vi "TimeTag_LSW_edits_oct28.vi"() -> ()   [LabVIEW 2015]
doc: "This sample project is built upon the standard state machine template and shows how you could create an application that acquires, analyzes, and presents data. It includes functionality for presenting configuration dialogs, preserving settings between executions, loading and saving data, as well as exporting graph images and text files.\n\nIt is most appropriate for data that is acquired instantly as it does not allow for screen updates mid acquisition nor does it allow for continuous streaming to disk."
uses:
  <vilib>/ptbypt/NI_PtbyPt.lvlib
panel:
  out "Channel 2&4 counts/sec":T1(graph)
  out "real coin cps 100 sec avg":dbl
  out "all coin cps":dbl
  out "real coin cps":dbl
  out "random coin cps":dbl
  out "Real coin cps":dbl(graph)
  out "total coin/sec - total random coin/sec":dbl
  out "total random coincidences/sec":dbl
  out "Total Coin per sec":dbl
  out "Ch2/4 coin/sec":dbl(graph)
  out "Ch2/4 Total Coincidences":dbl
  out "Channel 2 CPS":dbl(graph)
  out "Channel 4 CPS":dbl(graph)
  out "Total Ch2 CPS":dbl
  out "Total Ch4 CPS":dbl
  in  "Averaging":dbl=10.0
  in  "Runs":dbl=100.0
  in  "Pulse TTL 2":bool
  in  "Pulse TTL 1":bool
  in  "Toggle\nTTL 2":bool
  in  "Toggle\nTTL 1":bool
  out "Total Starts":dbl
  in  "Record data":bool
  out "Initial time":dbl
  out "Elapsed time (s)":dbl
  out "FPGA_Run Status":dbl
  out "USB_Open Status":dbl
  out "Channel 4 Total\nCounts":dbl
  out "Channel 3 Total\nCounts":dbl
  out "Channel 2 Total\nCounts":dbl
  out "Channel 1 Total\nCounts":dbl
  in  "File Name":string="C:\\FPGA\\test.txt"
  out "?":dbl
  out "?":dbl
  out "?":dbl
  out "?":dbl
  out "stats":i64[](array[numeric])
  in  "Stop":bool
  out "Channel 4 CPS":dbl(knob) scale=0.0..2000000.0
  out "Channel 3 CPS":dbl(knob) scale=0.0..600.0
  out "Channel 2 CPS":dbl(knob) scale=0.0..700.0
  out "Channel 1 CPS":dbl(knob) scale=0.0..600.0
  # "Starts"
  # "Channel 1"
  # "Channel 2"
  # "Channel 3"
  # "Channel 4"
  # "Coincidence Channels 1 & 2"
  # "Coincidence Channels 1 & 3"
  # "Coincidence Channels 1 & 4"
  # "Coincidence Channels 2 & 3"
  # "Coincidence Channels 2 & 4"
  # "Coincidence Channels 3 & 4"
  # "Coincidence Channels 1 & 2 & 3"
  # "Coincidence Channels 1 & 2 & 4"
  # "Coincidence Channels 1 & 3 & 4"
  # "Coincidence Channels 2 & 3 & 4"
  # "C:\\FPGA_Lauren"
  # "Coincidence Channels 1 & 2 & 3 & 4"
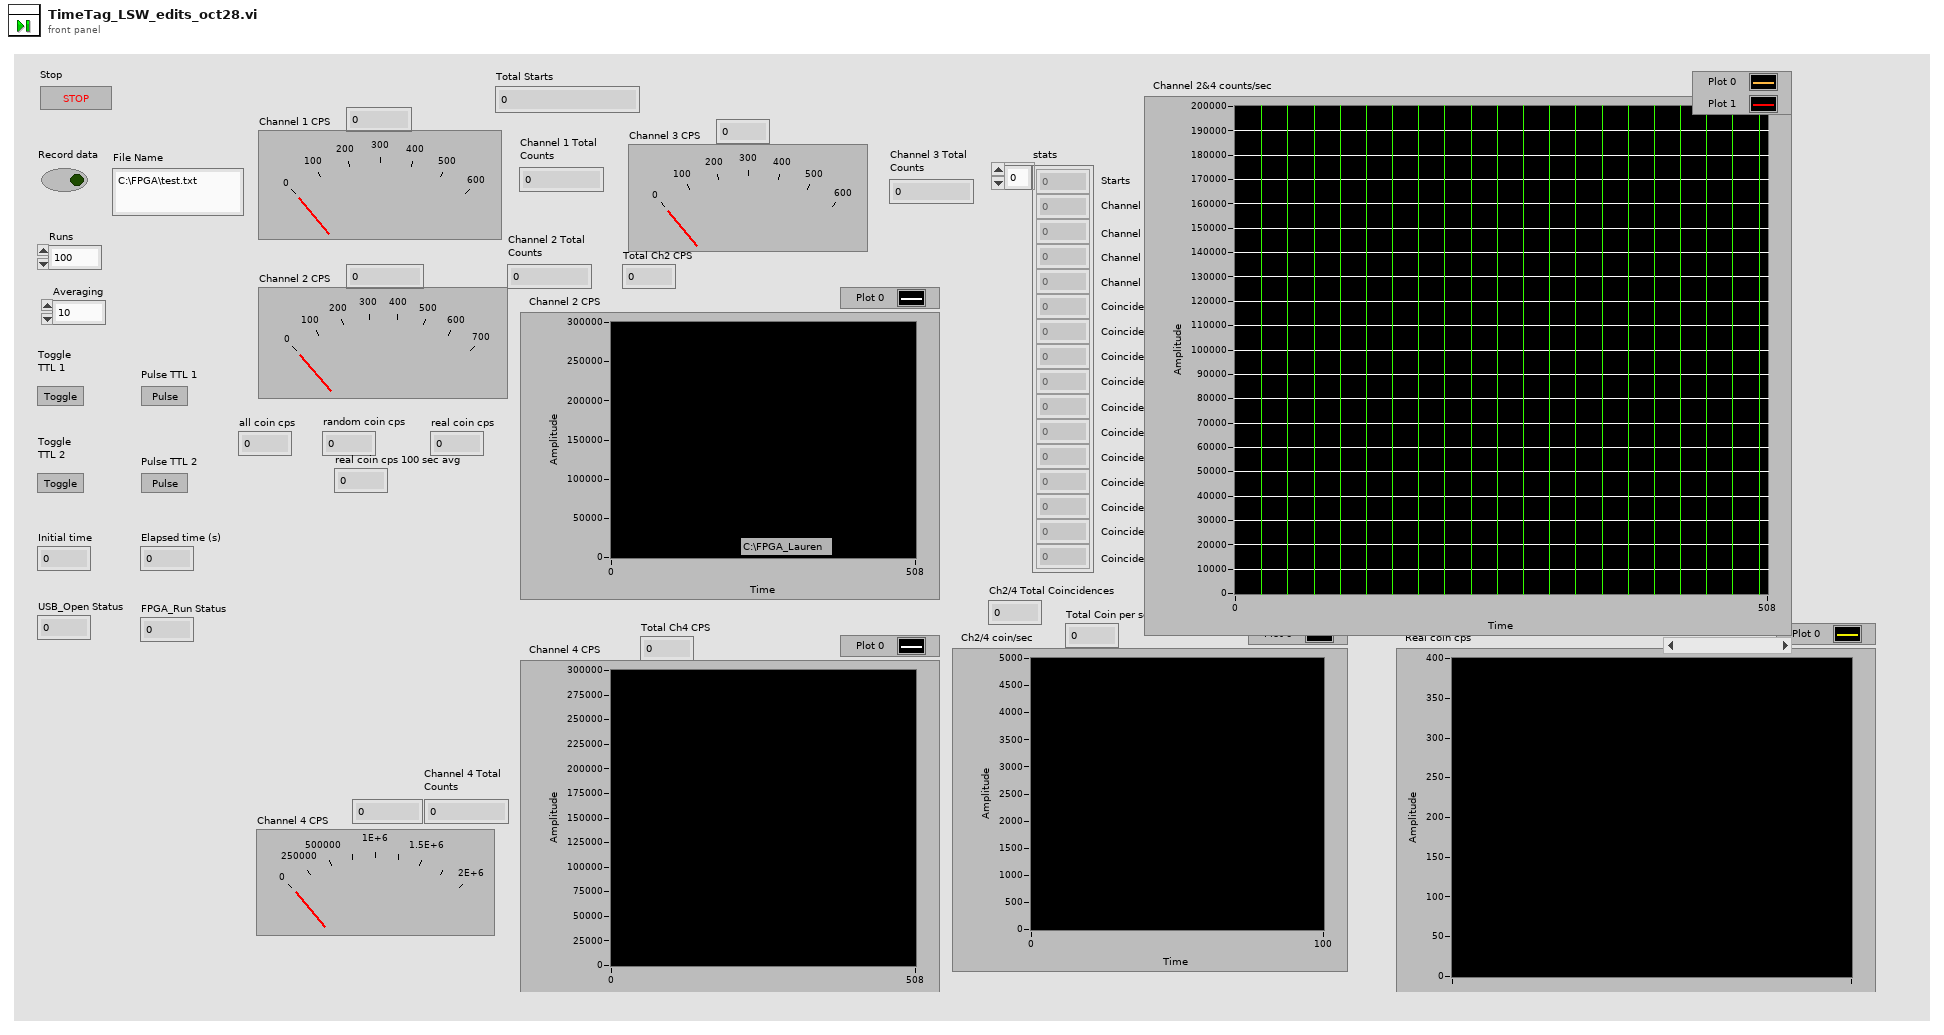
[diagram p1: front panel]
types:
  T1 = cluster{"[0]":dbl, "[1]":dbl, "[2]":dbl, "[3]":dbl, "[4]":dbl, "[5]":dbl, "[6]":dbl, "[7]":dbl, "[8]":dbl}
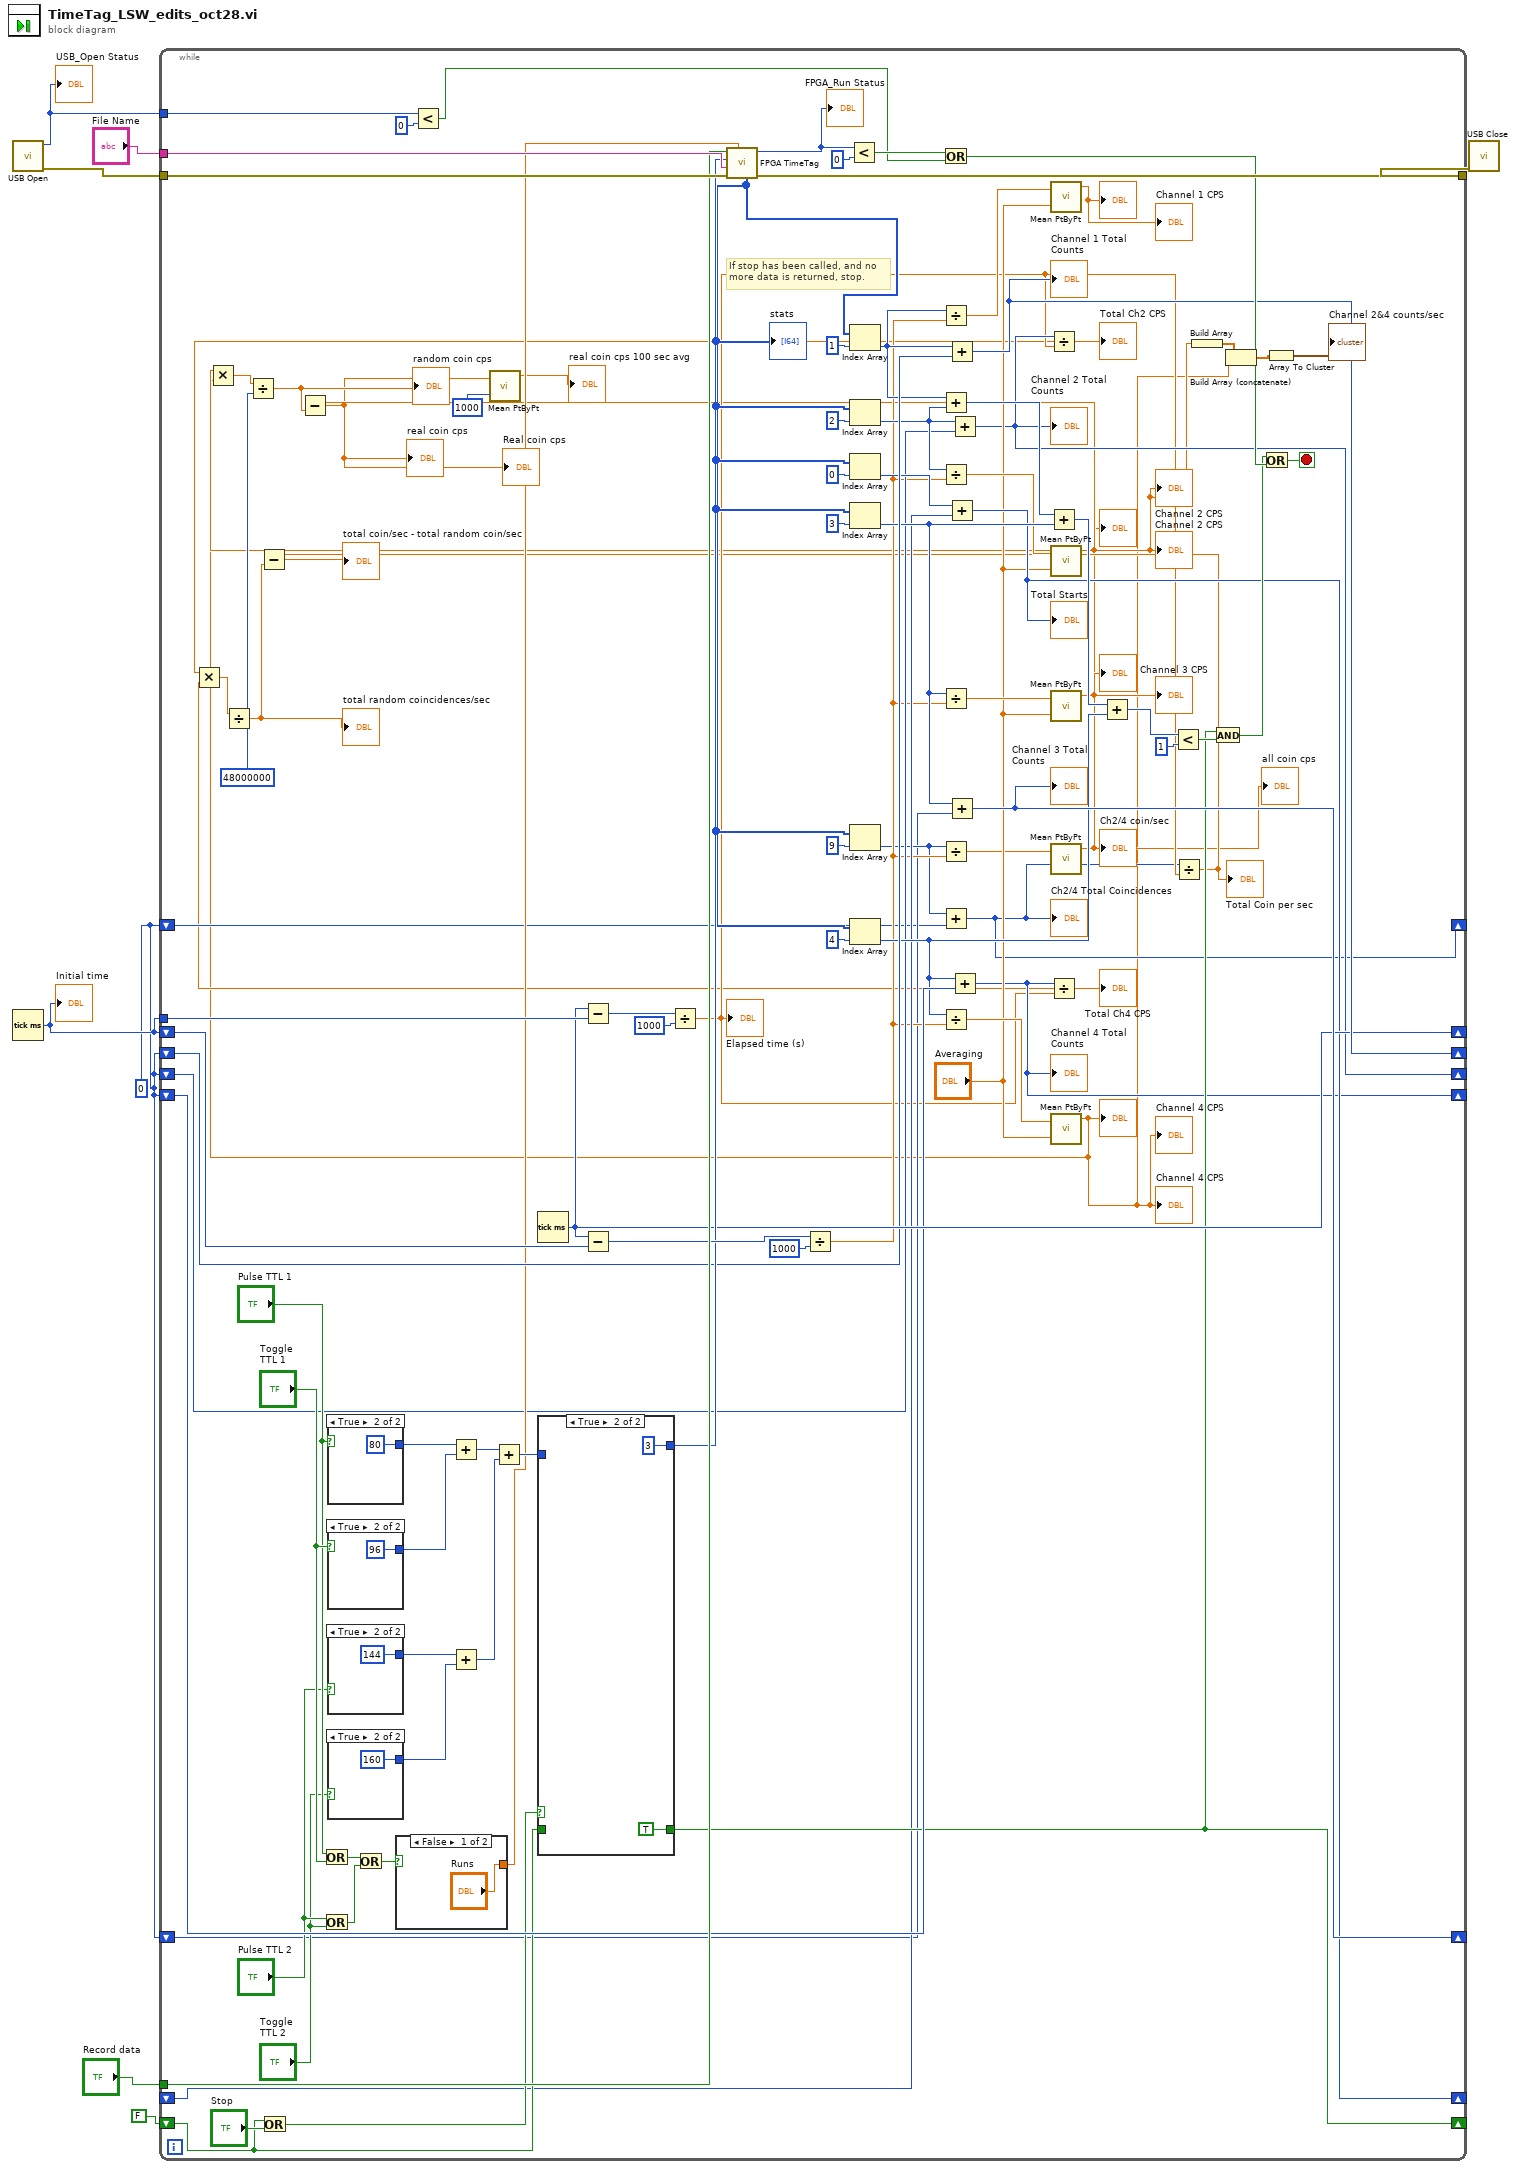
[diagram p0: block diagram]
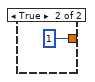
[diagram p2: hidden frame]
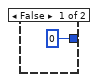
[diagram p3: hidden frame]
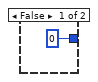
[diagram p4: hidden frame]
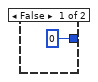
[diagram p5: hidden frame]
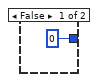
[diagram p6: hidden frame]
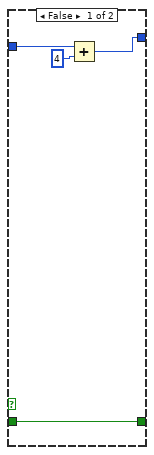
[diagram p7: hidden frame]
diagram:
  w1 = 0
  n1 = call "USB Open.vi"() -> ("error out"=w6:errorcluster, "function return"=w3:i32)  [unwired: 10 in]
  "USB_Open Status" <- w3
  n2 = Tick Count (ms)() -> (millisecond timer value=w4:u32)
  "Initial time" <- w4
  n3 = while {
    tunnel: w4 -> [w106]
    shift-right: [w84] -> _
    shift-left: w1 -> [w80]
    shift-right: [w38] -> _
    shift-left: w1 -> [w34]
    shift-right: [w83] -> _
    shift-left: w1 -> [w30]
    shift-right: [w39] -> _
    shift-left: w1 -> [w79]
    tunnel: w6 -> [w96]
    tunnel: [w97] -> w5
    tunnel: "Record data" -> [w94]
    tunnel: "File Name" -> [w95]
    shift-right: [w81] -> _
    shift-left: w4 -> [w92]
    tunnel: w3 -> [w88]
    shift-right: [w68] -> _
    shift-left: FALSE -> [w65]
    shift-right: [w61] -> _
    shift-left: _ -> [w62]
    shift-right: [w27] -> _
    shift-left: w1 -> [w29]
    stop <- w98 stop-if-true
    w21 = 48000000
    # "If stop has been called, and no\nmore data is returned, stop."
    n4 = Or(x=w65, y="Stop") -> (x .or. y?=w67:bool)
    n5 = Or(x="Pulse TTL 1", y="Toggle\nTTL 1") -> (x .or. y?=w52:bool)
    n6 = Or(x="Pulse TTL 2", y="Toggle\nTTL 2") -> (x .or. y?=w53:bool)
    n7 = case shown="True" "Pulse TTL 1" {
      tunnel: [0 80] -> w60
      frame False {
      }
      frame True {
      }
    }
    n8 = case shown="True" "Toggle\nTTL 1" {
      tunnel: [0 96] -> w59
      frame False {
      }
      frame True {
      }
    }
    n9 = case shown="True" "Pulse TTL 2" {
      tunnel: [0 144] -> w56
      frame False {
      }
      frame True {
      }
    }
    n10 = case shown="True" "Toggle\nTTL 2" {
      tunnel: [0 160] -> w57
      frame False {
      }
      frame True {
      }
    }
    n11 = Or(x=w52, y=w53) -> (x .or. y?=w54:bool)
    n12 = case shown="False" w54 {
      tunnel: ["Runs" 1] -> w50
      frame False {
      }
      frame True {
      }
    }
    n13 = Less?(x=w88, y=0) -> (x < y?=w86:bool)
    n14 = Add(x=w60, y=w59) -> (x+y=w58:i32)
    n15 = Add(x=w56, y=w57) -> (x+y=w55:i32)
    n16 = Add(x=w58, y=w55) -> (x+y=w51:i32)
    n17 = Tick Count (ms)() -> (millisecond timer value=w81:u32)
    n18 = case shown="True" w67 {
      tunnel: [w118 3] -> w82
      tunnel: [w120 TRUE] -> w68
      tunnel: w65 -> [w120 _]
      tunnel: w51 -> [w117 _]
      frame False {
        n19 = Add(x=w117, y=4) -> (x+y=w118:i32)
      }
      frame True {
      }
    }
    n20 = Subtract(x=w81, y=w106) -> (x-y=w105:u32)
    n21 = Subtract(x=w81, y=w92) -> (x-y=w91:u32)
    n22 = Divide(x=w105, y=1000) -> (x/y=w28:dbl)
    "Elapsed time (s)" <- w28
    n23 = call "FPGA TimeTag.vi"("runs"=w50, "error in (no error)"=w96, "fileName"=w95, "fpgaCommand"=w82, "saveData"=w94) -> ("error out"=w97:errorcluster, "function return"=w93:i32, "stats"=w36:i64[])  [unwired: 4 in]
    "stats" <- w36
    "FPGA_Run Status" <- w93
    n24 = Divide(x=w91, y=1000) -> (x/y=w33:dbl)
    n25 = Less?(x=w93, y=0) -> (x < y?=w87:bool)
    n26 = Index Array(array=w36, index=1) -> (element=w71:i64)
    n27 = Index Array(array=w36, index=2) -> (element=w78:i64)
    n28 = Index Array(array=w36, index=0) -> (element=w63:i64)
    n29 = Index Array(array=w36, index=3) -> (element=w74:i64)
    n30 = Index Array(array=w36, index=9) -> (element=w31:i64)
    n31 = Index Array(array=w36, index=4) -> (element=w75:i64)
    n32 = Or(x=w87, y=w86) -> (x .or. y?=w85:bool)
    n33 = Divide(x=w71, y=w33) -> (x/y=w45:dbl)
    n34 = Add(x=w71, y=w78) -> (x+y=w73:i64)
    n35 = Divide(x=w78, y=w33) -> (x/y=w44:dbl)
    n36 = Divide(x=w74, y=w33) -> (x/y=w43:dbl)
    n37 = Divide(x=w31, y=w33) -> (x/y=w32:dbl)
    n38 = Add(x=w31, y=w29) -> (x+y=w27:i64)
    "Ch2/4 Total Coincidences" <- w27
    n39 = Divide(x=w75, y=w33) -> (x/y=w41:dbl)
    n40 = Add(x=w71, y=w80) -> (x+y=w84:i64)
    "Channel 1 Total\nCounts" <- w84
    n41 = Add(x=w63, y=w62) -> (x+y=w61:i64)
    "Total Starts" <- w61
    n42 = Add(x=w74, y=w30) -> (x+y=w83:i64)
    "Channel 3 Total\nCounts" <- w83
    n43 = Add(x=w78, y=w34) -> (x+y=w38:i64)
    "Channel 2 Total\nCounts" <- w38
    n44 = Add(x=w75, y=w79) -> (x+y=w39:i64)
    "Channel 4 Total\nCounts" <- w39
    n45 = Divide(x=w38, y=w28) -> (x/y=w24:dbl)
    "Total Ch2 CPS" <- w24
    n46 = Add(x=w73, y=w74) -> (x+y=w77:i64)
    n47 = Divide(x=w39, y=w28) -> (x/y=w23:dbl)
    "Total Ch4 CPS" <- w23
    n48 = Multiply(x=w24, y=w23) -> (x*y=w22:dbl)
    n49 = Divide(x=w22, y=w21) -> (x/y=w25:dbl)
    "total random coincidences/sec" <- w25
    n50 = call <vilib>:"Mean PtByPt.vi"("x"=w45, "sample length"="Averaging") -> ("mean"=→"Channel 1 CPS" →"?":dbl)  [unwired: 2 in, 1 out]
    n51 = call <vilib>:"Mean PtByPt.vi"("x"=w44, "sample length"="Averaging") -> ("mean"=w13:dbl)  [unwired: 2 in, 1 out]
    "Channel 2 CPS" <- w13
    "?" <- w13
    "Channel 2 CPS" <- w13
    n52 = call <vilib>:"Mean PtByPt.vi"("x"=w43, "sample length"="Averaging") -> ("mean"=→"Channel 3 CPS" →"?":dbl)  [unwired: 2 in, 1 out]
    n53 = call <vilib>:"Mean PtByPt.vi"("x"=w32) -> ("mean"=w17:dbl)  [unwired: 3 in, 1 out]
    "Ch2/4 coin/sec" <- w17
    "all coin cps" <- w17
    n54 = call <vilib>:"Mean PtByPt.vi"("x"=w41, "sample length"="Averaging") -> ("mean"=w11:dbl)  [unwired: 2 in, 1 out]
    "Channel 4 CPS" <- w11
    "?" <- w11
    "Channel 4 CPS" <- w11
    n55 = Multiply(x=w13, y=w11) -> (x*y=w20:dbl)
    n56 = Divide(x=w20, y=w21) -> (x/y=w19:dbl)
    "random coin cps" <- w19
    n57 = Subtract(x=w17, y=w19) -> (x-y=w16:dbl)
    "Real coin cps" <- w16
    "real coin cps" <- w16
    n58 = call <vilib>:"Mean PtByPt.vi"("x"=w16, "sample length"=1000) -> ("mean"=→"real coin cps 100 sec avg":dbl)  [unwired: 2 in, 1 out]
    n59 = Add(x=w77, y=w75) -> (x+y=w76:i64)
    n60 = Less?(x=w76, y=1) -> (x < y?=w70:bool)
    n61 = Divide(x=w27, y=w28) -> (x/y=w26:dbl)
    "Total Coin per sec" <- w26
    n62 = Subtract(x=w26, y=w25) -> (x-y=→"total coin/sec - total random coin/sec":dbl)
    n63 = Build Array(w13) -> (w12:dbl[])
    n64 = And(x=w68, y=w70) -> (x .and. y?=w69:bool)
    n65 = Build Array (concatenate)(w12, w11) -> (w10:dbl[])
    n66 = Or(x=w69, y=w85) -> (x .or. y?=w98:bool)
    n67 = Array To Cluster(array=w10) -> (cluster=→"Channel 2&4 counts/sec":T1)
  }
  n68 = call "USB Close.vi"("error in (no error)"=w5) -> ()  [unwired: 9 in, 2 out]
